vi "YCursorSlider.vi"(5 "Current Trans":u16, 6 "Force Include Focus?":bool=TRUE, 7 "Cursor\nHold-off":dbl, 8 "Dual XDCR Settings":T1 {"XDCR Settings"."UT340 Controls"."Low Pass Filter (MHz)" min=-6 max=60 step=1; "XDCR Settings"."UT340 Controls"."High Pass Filter (MHz)" min=1 max=20 step=1; "XDCR Settings"."UT340 Controls"."Rep Rate (Hz)" min=20 step=1; "XDCR Settings"."UT340 Controls"."Pulse Width (ns)" min=100.0 max=250.0 step=2.0; "XDCR Settings"."UT340 Controls"."Voltage" min=100 max=250 step=2; "XDCR Settings"."UT340 Controls"."PC Gain (dB)" min=2 max=72; "XDCR Settings"."UT340 Controls"."PE Gain (dB)" min=-6 max=60 step=1; "XDCR Settings"."JSR Complete"."JSR Trigger Settings"."PRF (Hz)" items=["100 Hz"=0.1, "200 Hz"=0.2, "400 Hz"=0.4, "600 Hz"=0.6, "800 Hz"=0.8, "1000 Hz"=1.0, "1250 Hz"=1.25, "1500 Hz"=1.5, "1750 Hz"=1.75, "2000 Hz"=2.0, "2500 Hz"=2.5, "3000 Hz"=3.0, "3500 Hz"=3.5, "4000 Hz"=4.0, "4500 Hz"=4.5, "5000 Hz"=5.0]; "XDCR Settings"."JSR Complete"."JSR Trigger Settings"."Trigger Source" items=["Internal", "External"]; "XDCR Settings"."JSR Complete"."JSR Trigger Settings"."External Trigger Limit" items=["No Limit", "5 kHz"]; "XDCR Settings"."JSR Complete"."JSR Receive Settings"."Gain (dB)" min=-13 max=66 step=1; "XDCR Settings"."JSR Complete"."JSR Receive Settings"."Low Pass Filter" items=["5 MHz"=5, "10 MHz"=10, "15 MHz"=15, "22.5 MHz"=22, "35 MHz"=35, "50 MHz"=50]; "XDCR Settings"."JSR Complete"."JSR Receive Settings"."High Pass Filter" items=["DC"=0, "1 MHz"=1000, "2.5 MHz"=2500, "5 MHz"=5000, "7.5 MHz"=7500, "12.5 MHz"=12500]; "XDCR Settings"."JSR Complete"."JSR Receive Settings"."Receiver Mode" items=["Echo", "Through"]; "XDCR Settings"."JSR Complete"."JSR Pulse Settings"."Pulser Voltage (V)" items=["100"=100, "125"=125, "150"=150, "175"=175, "200"=200, "225"=225, "250"=250, "275"=275, "300"=300, "325"=325, "350"=350, "375"=375, "400"=400, "425"=425, "450"=450, "475"=475]; "XDCR Settings"."JSR Complete"."JSR Pulse Settings"."Pulser Impedance" items=["High z", "Low z"]; "XDCR Settings"."JSR Complete"."JSR Pulse Settings"."Pulse Energy Level" items=["0 (Minimum)", "1", "2", "3 (Maximum)"]; "XDCR Settings"."JSR Complete"."JSR Pulse Settings"."Damping" items=["331 Ohms"=331, "198 Ohms"=198, "142 Ohms"=142, "110 Ohms"=110, "92 Ohms"=92, "77 Ohms"=77, "67 Ohms"=67, "59 Ohms"=59, "52 Ohms"=52, "47 Ohms"=47, "43 Ohms"=43, "39 Ohms"=39, "37 Ohms"=37, "34 Ohms"=34, "32 Ohms"=32, "30 Ohms"=30]; "XDCR Settings"."Panametrics Settings"."FINE ATTENUATION" items=["00.0", "00.5", "01.0", "01.5", "02.0", "02.5", "03.0", "03.5", "04.0", "04.5", "05.0", "05.5", "06.0", "06.5", "07.0", "07.5", "08.0", "08.5", "09.0", "09.5", "10.0", "10.5", "11.0", "11.5", "12.0", "12.5", "13.0", "13.5", "14.0", "14.5", "15.0", "15.5"]; "XDCR Settings"."Panametrics Settings"."COARSE ATTENUATION" items=["00.0", "10.0", "20.0", "30.0", "40.0", "50.0"]; "XDCR Settings"."Panametrics Settings"."GAIN (db)" items=["26.0", "40.0", "54.0"]; "XDCR Settings"."Panametrics Settings"."PRF (KHz)" items=["XREMT", "EXBNC", "0.200", "0.500", "1.000", "2.000", "5.000", "10.00", "20.00"]; "XDCR Settings"."Panametrics Settings"."MODE" items=["P/ E", "THRU", "RPP", "EXT_PLSR"]; "XDCR Settings"."Panametrics Settings"."LP FILT (MHz)" items=["20", "50", "100", "200"]; "XDCR Settings"."Panametrics Settings"."HP FILT (KHz)" items=["1", "1000", "3000", "10000"]; "XDCR Settings"."Panametrics Settings"."DAMPING (Ohm)" items=["7", "10", "16", "20", "26", "30", "40", "50"]; "XDCR Settings"."Panametrics Settings"."ENERGY (uJ)" items=["1", "2", "4", "8", "16", "32"]; "XDCR Settings"."Daxsonics Settings"."Freq (MHz)" items=["4"=4, "5"=5, "6"=6, "8"=8, "10"=10, "12"=12, "14"=14, "15"=15, "16"=16, "17"=17, "18"=18, "20"=20, "25"=25, "30"=30, "35"=35, "40"=40, "45"=45, "50"=50]; "XDCR Settings"."Daxsonics Settings"."Voltage (V)" items=["0"=0, "5"=5, "10"=10, "15"=15, "20"=20, "25"=25, "30"=30, "35"=35, "40"=40, "45"=45, "50"=50, "55"=55, "60"=60, "65"=65, "70"=70, "75"=75, "80"=80, "85"=85, "90"=90, "95"=95, "100"=100, "110"=110, "120"=120, "130"=130, "140"=140, "150"=150, "160"=160, "170"=170, "180"=180, "190"=190]; "XDCR Settings"."Daxsonics Settings"."Gain (dB)" items=["22"=22, "25"=25, "28"=28, "31"=31, "34"=34, "37"=37, "40"=40, "43"=43, "46"=46, "49"=49, "52"=52, "55"=55, "58"=58, "61"=61, "64"=64, "67"=67]; "XDCR Settings"."Digitizer Settings"."Additional dig delay (ms)" format="%.2f"; "XDCR Settings"."Digitizer Settings"."Time scale per Div" items=["100 ns"=0.1, "200 ns"=0.2, "500 ns"=0.5, "1 micros"=1.0, "2 micros"=2.0, "5 micros"=5.0, "10 micros"=10.0, "20 micros"=20.0, "50 micros"=50.0, "100 micros"=100.0, "200 micros"=200.0, "500 micros"=500.0, "1 ms"=1000.0, "2 ms"=2000.0, "5 ms"=5000.0, "10 ms"=10000.0, "20 ms"=20000.0, "50 ms"=50000.0, "100 ms"=100000.0, "200 ms"=200000.0]; "XDCR Settings"."Digitizer Settings"."RF data Sampling"."rf points per line" min=1; "XDCR Settings"."Digitizer Settings"."RF data Sampling"."Ref Delay (ms)" format="%.2f"}, 9 "CtlRef":refnum<vi>) -> (1 "Z Scan Size":dbl, 2 "Dual XDCR Settings out":T1 {"XDCR Settings"."UT340 Controls"."Low Pass Filter (MHz)" min=-6 max=60 step=1; "XDCR Settings"."UT340 Controls"."High Pass Filter (MHz)" min=1 max=20 step=1; "XDCR Settings"."UT340 Controls"."Rep Rate (Hz)" min=20 step=1; "XDCR Settings"."UT340 Controls"."Pulse Width (ns)" min=100.0 max=250.0 step=2.0; "XDCR Settings"."UT340 Controls"."Voltage" min=100 max=250 step=2; "XDCR Settings"."UT340 Controls"."PC Gain (dB)" min=2 max=72; "XDCR Settings"."UT340 Controls"."PE Gain (dB)" min=-6 max=60 step=1; "XDCR Settings"."JSR Complete"."JSR Trigger Settings"."PRF (Hz)" items=["100 Hz"=0.1, "200 Hz"=0.2, "400 Hz"=0.4, "600 Hz"=0.6, "800 Hz"=0.8, "1000 Hz"=1.0, "1250 Hz"=1.25, "1500 Hz"=1.5, "1750 Hz"=1.75, "2000 Hz"=2.0, "2500 Hz"=2.5, "3000 Hz"=3.0, "3500 Hz"=3.5, "4000 Hz"=4.0, "4500 Hz"=4.5, "5000 Hz"=5.0]; "XDCR Settings"."JSR Complete"."JSR Trigger Settings"."Trigger Source" items=["Internal", "External"]; "XDCR Settings"."JSR Complete"."JSR Trigger Settings"."External Trigger Limit" items=["No Limit", "5 kHz"]; "XDCR Settings"."JSR Complete"."JSR Receive Settings"."Gain (dB)" min=-13 max=66 step=1; "XDCR Settings"."JSR Complete"."JSR Receive Settings"."Low Pass Filter" items=["5 MHz"=5, "10 MHz"=10, "15 MHz"=15, "22.5 MHz"=22, "35 MHz"=35, "50 MHz"=50]; "XDCR Settings"."JSR Complete"."JSR Receive Settings"."High Pass Filter" items=["DC"=0, "1 MHz"=1000, "2.5 MHz"=2500, "5 MHz"=5000, "7.5 MHz"=7500, "12.5 MHz"=12500]; "XDCR Settings"."JSR Complete"."JSR Receive Settings"."Receiver Mode" items=["Echo", "Through"]; "XDCR Settings"."JSR Complete"."JSR Pulse Settings"."Pulser Voltage (V)" items=["100"=100, "125"=125, "150"=150, "175"=175, "200"=200, "225"=225, "250"=250, "275"=275, "300"=300, "325"=325, "350"=350, "375"=375, "400"=400, "425"=425, "450"=450, "475"=475]; "XDCR Settings"."JSR Complete"."JSR Pulse Settings"."Pulser Impedance" items=["High z", "Low z"]; "XDCR Settings"."JSR Complete"."JSR Pulse Settings"."Pulse Energy Level" items=["0 (Minimum)", "1", "2", "3 (Maximum)"]; "XDCR Settings"."JSR Complete"."JSR Pulse Settings"."Damping" items=["331 Ohms"=331, "198 Ohms"=198, "142 Ohms"=142, "110 Ohms"=110, "92 Ohms"=92, "77 Ohms"=77, "67 Ohms"=67, "59 Ohms"=59, "52 Ohms"=52, "47 Ohms"=47, "43 Ohms"=43, "39 Ohms"=39, "37 Ohms"=37, "34 Ohms"=34, "32 Ohms"=32, "30 Ohms"=30]; "XDCR Settings"."Panametrics Settings"."FINE ATTENUATION" items=["00.0", "00.5", "01.0", "01.5", "02.0", "02.5", "03.0", "03.5", "04.0", "04.5", "05.0", "05.5", "06.0", "06.5", "07.0", "07.5", "08.0", "08.5", "09.0", "09.5", "10.0", "10.5", "11.0", "11.5", "12.0", "12.5", "13.0", "13.5", "14.0", "14.5", "15.0", "15.5"]; "XDCR Settings"."Panametrics Settings"."COARSE ATTENUATION" items=["00.0", "10.0", "20.0", "30.0", "40.0", "50.0"]; "XDCR Settings"."Panametrics Settings"."GAIN (db)" items=["26.0", "40.0", "54.0"]; "XDCR Settings"."Panametrics Settings"."PRF (KHz)" items=["XREMT", "EXBNC", "0.200", "0.500", "1.000", "2.000", "5.000", "10.00", "20.00"]; "XDCR Settings"."Panametrics Settings"."MODE" items=["P/ E", "THRU", "RPP", "EXT_PLSR"]; "XDCR Settings"."Panametrics Settings"."LP FILT (MHz)" items=["20", "50", "100", "200"]; "XDCR Settings"."Panametrics Settings"."HP FILT (KHz)" items=["1", "1000", "3000", "10000"]; "XDCR Settings"."Panametrics Settings"."DAMPING (Ohm)" items=["7", "10", "16", "20", "26", "30", "40", "50"]; "XDCR Settings"."Panametrics Settings"."ENERGY (uJ)" items=["1", "2", "4", "8", "16", "32"]; "XDCR Settings"."Daxsonics Settings"."Freq (MHz)" items=["4"=4, "5"=5, "6"=6, "8"=8, "10"=10, "12"=12, "14"=14, "15"=15, "16"=16, "17"=17, "18"=18, "20"=20, "25"=25, "30"=30, "35"=35, "40"=40, "45"=45, "50"=50]; "XDCR Settings"."Daxsonics Settings"."Voltage (V)" items=["0"=0, "5"=5, "10"=10, "15"=15, "20"=20, "25"=25, "30"=30, "35"=35, "40"=40, "45"=45, "50"=50, "55"=55, "60"=60, "65"=65, "70"=70, "75"=75, "80"=80, "85"=85, "90"=90, "95"=95, "100"=100, "110"=110, "120"=120, "130"=130, "140"=140, "150"=150, "160"=160, "170"=170, "180"=180, "190"=190]; "XDCR Settings"."Daxsonics Settings"."Gain (dB)" items=["22"=22, "25"=25, "28"=28, "31"=31, "34"=34, "37"=37, "40"=40, "43"=43, "46"=46, "49"=49, "52"=52, "55"=55, "58"=58, "61"=61, "64"=64, "67"=67]; "XDCR Settings"."Digitizer Settings"."Additional dig delay (ms)" format="%.2f"; "XDCR Settings"."Digitizer Settings"."Time scale per Div" items=["100 ns"=0.1, "200 ns"=0.2, "500 ns"=0.5, "1 micros"=1.0, "2 micros"=2.0, "5 micros"=5.0, "10 micros"=10.0, "20 micros"=20.0, "50 micros"=50.0, "100 micros"=100.0, "200 micros"=200.0, "500 micros"=500.0, "1 ms"=1000.0, "2 ms"=2000.0, "5 ms"=5000.0, "10 ms"=10000.0, "20 ms"=20000.0, "50 ms"=50000.0, "100 ms"=100000.0, "200 ms"=200000.0]; "XDCR Settings"."Digitizer Settings"."RF data Sampling"."rf points per line" min=1; "XDCR Settings"."Digitizer Settings"."RF data Sampling"."Ref Delay (ms)" format="%.2f"})   [LabVIEW 2022 SP3]
uses:
  ScanningControl/DualXDCR/Dual XDCR Complete Settings.ctl
  ScanningControl/DualXDCR/XDCRSettings.ctl
  ScanningControl/Pulsers/Daxsonics/-DaxSubroutines/Dax_Control_Cluster.ctl
  ScanningControl/Pulsers/Panametrics/Pana5900.ctl
  ScanningControl/Pulsers/JSR/Controls/JSR Complete.ctl
  ScanningControl/Pulsers/JSR/Controls/JSR Pulse.ctl
  ScanningControl/Pulsers/JSR/Controls/Damping.ctl
  ScanningControl/Pulsers/JSR/Controls/Energy.ctl
  ScanningControl/Pulsers/JSR/Controls/Z.ctl
  ScanningControl/Pulsers/JSR/Controls/Volt.ctl
  ScanningControl/Pulsers/JSR/Controls/JSR Recieve.ctl
  ScanningControl/Pulsers/JSR/Controls/Mode.ctl
  ScanningControl/Pulsers/JSR/Controls/HPF.ctl
  ScanningControl/Pulsers/JSR/Controls/LPF.ctl
  ScanningControl/Pulsers/JSR/Controls/Gain.ctl
  ScanningControl/Pulsers/JSR/Controls/JSR Trigger.ctl
  ScanningControl/Pulsers/JSR/Controls/Trig Limit.ctl
  ScanningControl/Pulsers/JSR/Controls/Trig Source.ctl
  ScanningControl/Pulsers/JSR/Controls/PRF.ctl
  ScanningControl/Pulsers/UTEX/Controls/UTEX Controls.ctl
  <vilib>/Analysis/baseanly.llb/Mean (DBL).vi
  Misc Programs/MathOperations/ModuloFraction.vi
  <vilib>/Analysis/NI_AALBase.lvlib
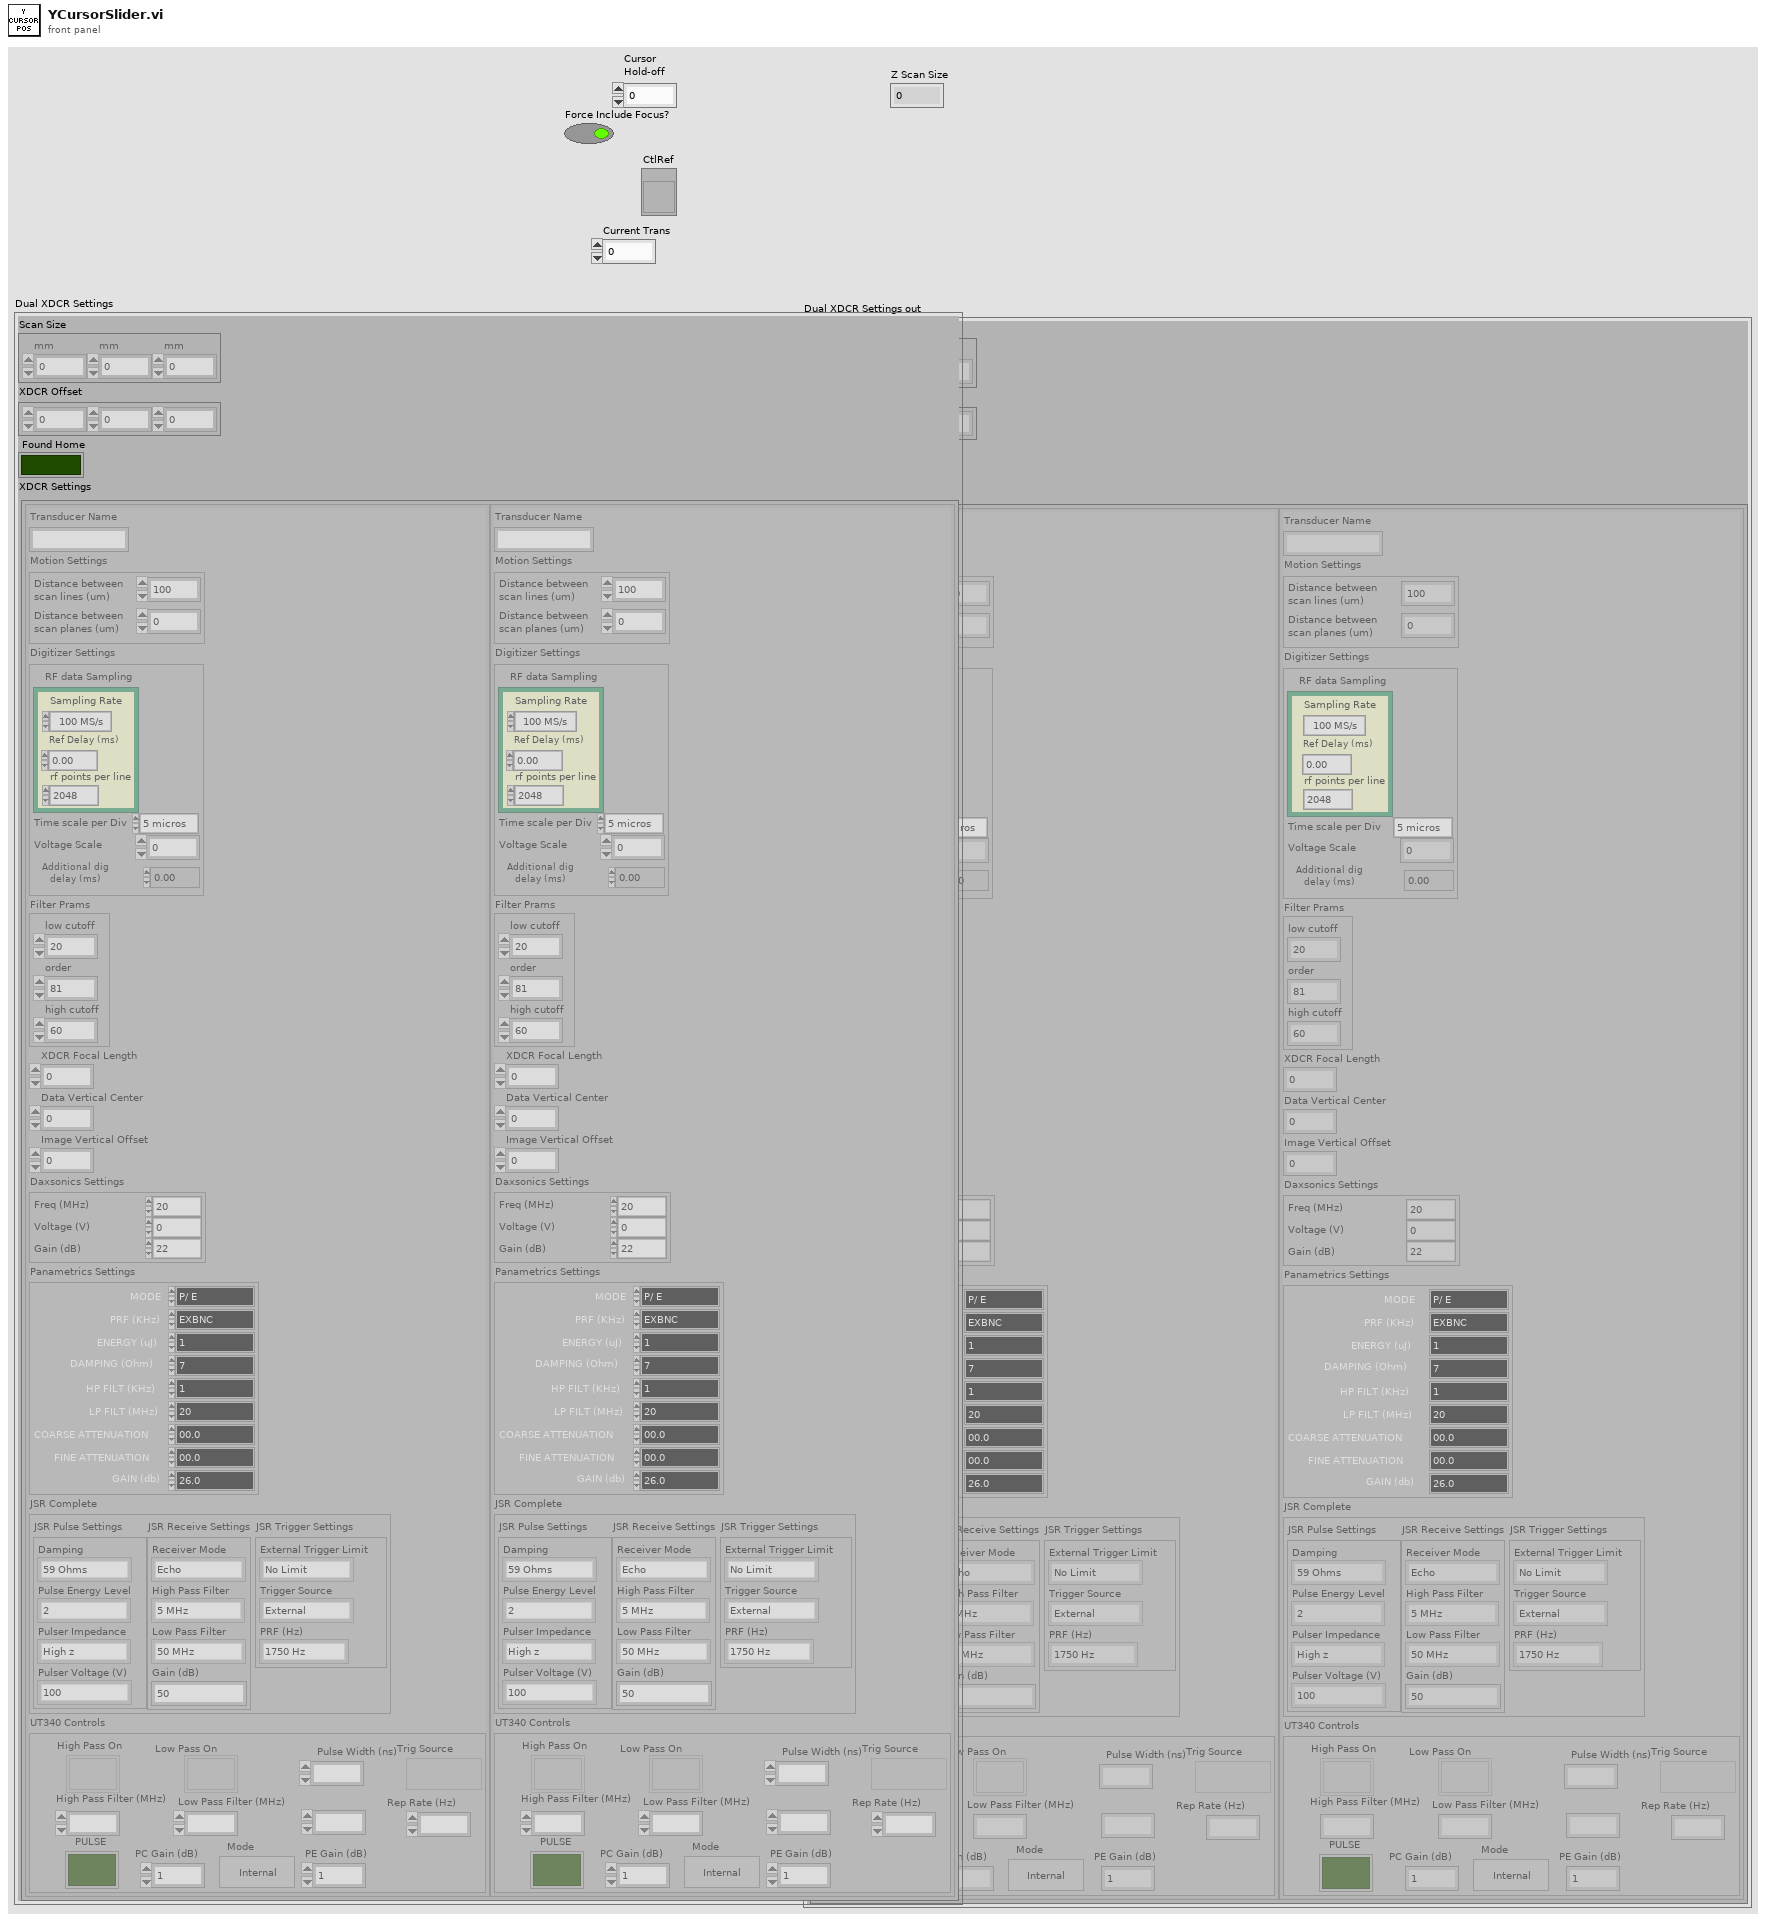
[diagram p1: front panel]
types:
  T1 = typedef "Dual XDCR Complete Settings.ctl" = cluster{"Scan Size":dbl[], "XDCR Offset":dbl[], "Found Home":bool, "XDCR Settings":T2[]}
  T2 = typedef "XDCRSettings.ctl" = cluster{"Transducer Name":string, "Motion Settings":cluster{"Distance between\nscan lines (um)":sgl, "Distance between\nscan planes (um)":sgl}, "Digitizer Settings":cluster{"RF data Sampling":cluster{"Sampling Rate":dbl, "Ref Delay (ms)":dbl, "rf points per line":i32}, "Time scale per Div":dbl, "Voltage Scale":dbl, "Additional dig delay (ms)":dbl}, "Filter Prams":cluster{"low cutoff":i32, "order":i32, "high cutoff":i32}, "XDCR Focal Length":dbl, "Data Vertical Center":dbl, "Image Vertical Offset":dbl, "Daxsonics Settings":T3, "Panametrics Settings":T4, "JSR Complete":T5, "UT340 Controls":T20}
  T3 = typedef "Dax_Control_Cluster.ctl" = cluster{"Freq (MHz) ":u16, "Voltage (V)":u16, "Gain (dB)":u16}
  T4 = typedef "Pana5900.ctl" = cluster{"ENERGY (uJ)":u16, "DAMPING (Ohm)":u16, "HP FILT (KHz) ":u16, "LP FILT (MHz)":u16, "MODE":u16, "PRF (KHz)":u16, "GAIN (db)":u16, "COARSE ATTENUATION":u16, "FINE ATTENUATION":u16}
  T5 = typedef "JSR Complete.ctl" = cluster{"JSR Pulse Settings":T6, "JSR Receive Settings":T11, "JSR Trigger Settings":T16}
  T6 = typedef "JSR Pulse.ctl" = cluster{"Damping":T7, "Pulse Energy Level":T8, "Pulser Impedance":T9, "Pulser Voltage (V)":T10}
  T7 = typedef "Damping.ctl" = i16
  T8 = typedef "Energy.ctl" = u16
  T9 = typedef "Z.ctl" = u16
  T10 = typedef "Volt.ctl" = i16
  T11 = typedef "JSR Recieve.ctl" = cluster{"Receiver Mode":T12, "High Pass Filter":T13, "Low Pass Filter":T14, "Gain (dB)":T15}
  T12 = typedef "Mode.ctl" = i8
  T13 = typedef "HPF.ctl" = u16
  T14 = typedef "LPF.ctl" = u16
  T15 = typedef "Gain.ctl" = i8
  T16 = typedef "JSR Trigger.ctl" = cluster{"External Trigger Limit":T17, "Trigger Source":T18, "PRF (Hz)":T19}
  T17 = typedef "Trig Limit.ctl" = i8
  T18 = typedef "Trig Source.ctl" = i8
  T19 = typedef "PRF.ctl" = dbl
  T20 = typedef "UTEX Controls.ctl" = cluster{"High Pass On":bool, "High Pass Filter (MHz)":i16, "Low Pass On":bool, "Low Pass Filter (MHz)":i16, "PE Gain (dB)":i16, "Voltage":i16, "Pulse Width (ns)":dbl, "Mode":bool, "PC Gain (dB)":i16, "Trig Source":bool, "Rep Rate (Hz)":i16, "PULSE":bool}
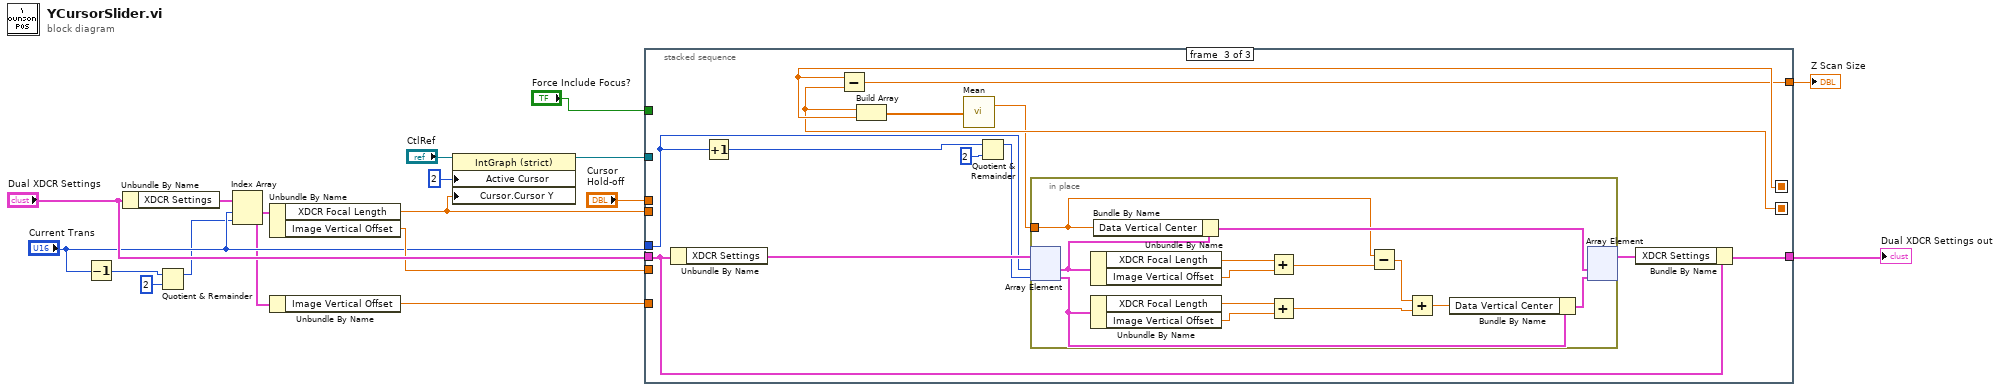
[diagram p0: block diagram]
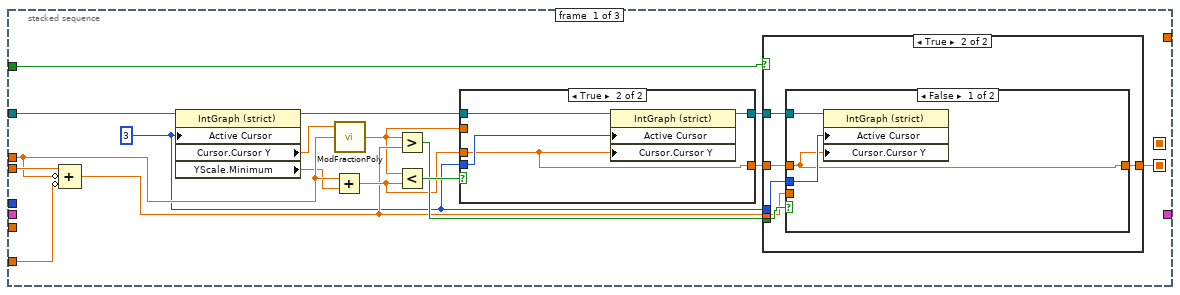
[diagram p2: hidden frame]
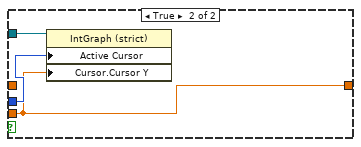
[diagram p4: hidden frame]
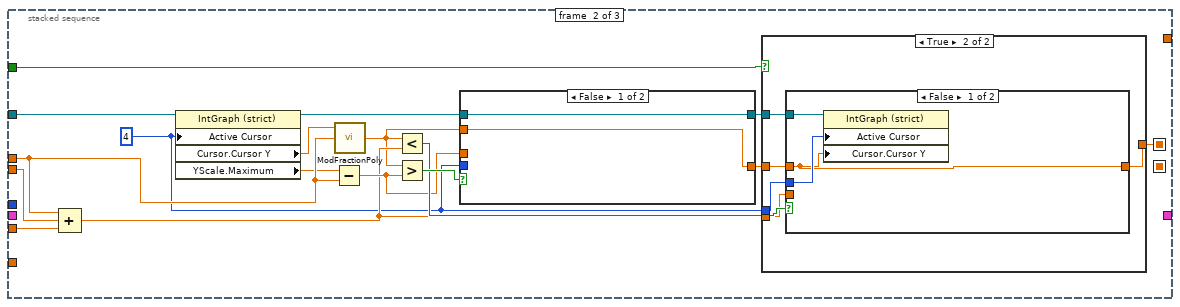
[diagram p6: hidden frame]
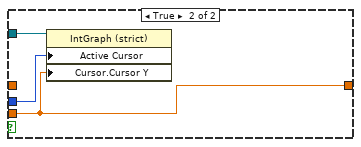
[diagram p8: hidden frame]
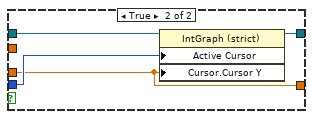
[diagram p9: hidden frame]
diagram:
  n1 = Decrement(x="Current Trans") -> (x-1=w1:u16)
  n2 = Unbundle By Name("Dual XDCR Settings") -> ("XDCR Settings"=w12:T2[])
  n3 = Quotient & Remainder(x=w1, y=u32 2) -> (x-y*floor(x/y)=w4:u32)  [unwired: 1 out]
  n4 = Index Array(array=w12, index #1="Current Trans", index #2=w4) -> (element #1=w13:T2, element #2=w3:T2)
  n5 = Unbundle By Name(w13) -> ("XDCR Focal Length"=w10:dbl, "Image Vertical Offset"=w7:dbl)
  n6 = Unbundle By Name(w3) -> ("Image Vertical Offset"=w2:dbl)
  n7 = property on="Property Node" class="IntGraph (strict)"(reference="CtlRef", "Active Cursor"=u32 2, "Cursor.Cursor Y"=w10) -> (reference out=w15:refnum<vi>)  [unwired: 1 in, 1 out]
  n8 = stacked-sequence {
    seq-local: [w33 _ _] -> [_ _ w94]
    seq-local: [_ w69 _] -> [_ _ w95]
    tunnel: w15 -> [w25 w61 _]
    tunnel: "Dual XDCR Settings" -> [_ _ w97]
    tunnel: "Current Trans" -> [_ _ w102]
    tunnel: w10 -> [w32 w68 _]
    tunnel: "Cursor\nHold-off" -> [w28 w65 _]
    tunnel: [_ _ w93] -> w17
    tunnel: [_ _ w92] -> w9
    tunnel: "Force Include Focus?" -> [w20 w56 _]
    tunnel: w7 -> [_ w55 _]
    tunnel: w2 -> [w19 _ _]
    frame #0 {
      w27 = u32 3 ("Active Cursor")
      n9 = Compound Arithmetic op=ADD(w32, invert w28, invert w19) -> (w30:dbl)
      n10 = property on="Property Node" class="IntGraph (strict)"(reference=w25, "Active Cursor"=w27) -> (reference out=w24:refnum<vi>, "Cursor.Cursor Y"=w26:dbl, "YScale.Minimum"=w23:dbl)  [unwired: 1 in, 1 out]
      n11 = Add(x=w28, y=w23) -> (x+y=w31:dbl)
      n12 = call-poly "ModFractionPoly.vi"("Modulo Fraction"=w28, "Input"=w26) -> ("Output"=w29:dbl)  [unwired: 1 in]
      n13 = Greater?(x=w29, y=w30) -> (0:w34:bool)
      n14 = Less?(x=w29, y=w31) -> (x < y?=w35:bool)
      n15 = case shown="True" w35 {
        tunnel: w24 -> [w49 w54]
        tunnel: [w50 w51] -> w22
        tunnel: w29 -> [w50 _]
        tunnel: w27 -> [_ w53]
        tunnel: w31 -> [_ w51]
        tunnel: [w49 w52] -> w21
        frame False {
        }
        frame True {
          n16 = property on="Property Node" class="IntGraph (strict)"(reference=w54, "Active Cursor"=w53, "Cursor.Cursor Y"=w51) -> (reference out=w52:refnum<vi>)  [unwired: 1 in, 1 out]
        }
      }
      n17 = case shown="True" w20 {
        tunnel: w34 -> [_ w42]
        tunnel: [w36 w41] -> w33
        tunnel: w30 -> [_ w40]
        tunnel: w27 -> [_ w39]
        tunnel: w22 -> [w36 w38]
        tunnel: w21 -> [_ w37]
        frame False {
        }
        frame True {
          n18 = case shown="False" w42 {
            tunnel: w37 -> [w45 w48]
            tunnel: w39 -> [w44 w47]
            tunnel: w40 -> [_ w46]
            tunnel: w38 -> [w43 _]
            tunnel: [w43 w46] -> w41
            frame False {
              n19 = property on="Property Node" class="IntGraph (strict)"(reference=w45, "Active Cursor"=w44, "Cursor.Cursor Y"=w43) -> ()  [unwired: 1 in, 2 out]
            }
            frame True {
              n20 = property on="Property Node" class="IntGraph (strict)"(reference=w48, "Active Cursor"=w47, "Cursor.Cursor Y"=w46) -> ()  [unwired: 1 in, 2 out]
            }
          }
        }
      }
    }
    frame #1 {
      w63 = u32 4 ("Active Cursor")
      n21 = Compound Arithmetic op=ADD(w65, w68, w55) -> (w66:dbl)
      n22 = property on="Property Node" class="IntGraph (strict)"(reference=w61, "Active Cursor"=w63) -> (reference out=w62:refnum<vi>, "Cursor.Cursor Y"=w60:dbl, "YScale.Maximum"=w59:dbl)  [unwired: 1 in, 1 out]
      n23 = Subtract(x=w59, y=w65) -> (x-y=w67:dbl)
      n24 = call-poly "ModFractionPoly.vi"("Modulo Fraction"=w65, "Input"=w60) -> ("Output"=w64:dbl)  [unwired: 1 in]
      n25 = Less?(x=w64, y=w66) -> (x < y?=w70:bool)
      n26 = Greater?(x=w64, y=w67) -> (0:w71:bool)
      n27 = case shown="False" w71 {
        tunnel: w62 -> [w85 w90]
        tunnel: [w86 w88] -> w58
        tunnel: w64 -> [w86 _]
        tunnel: w63 -> [_ w89]
        tunnel: w67 -> [_ w88]
        tunnel: [w85 w87] -> w57
        frame False {
        }
        frame True {
          n28 = property on="Property Node" class="IntGraph (strict)"(reference=w90, "Active Cursor"=w89, "Cursor.Cursor Y"=w88) -> (reference out=w87:refnum<vi>)  [unwired: 1 in, 1 out]
        }
      }
      n29 = case shown="True" w56 {
        tunnel: w70 -> [_ w78]
        tunnel: [w72 w77] -> w69
        tunnel: w66 -> [_ w76]
        tunnel: w63 -> [_ w75]
        tunnel: w58 -> [w72 w74]
        tunnel: w57 -> [_ w73]
        frame False {
        }
        frame True {
          n30 = case shown="False" w78 {
            tunnel: w73 -> [w81 w84]
            tunnel: w75 -> [w80 w83]
            tunnel: w76 -> [_ w82]
            tunnel: w74 -> [w79 _]
            tunnel: [w79 w82] -> w77
            frame False {
              n31 = property on="Property Node" class="IntGraph (strict)"(reference=w81, "Active Cursor"=w80, "Cursor.Cursor Y"=w79) -> ()  [unwired: 1 in, 2 out]
            }
            frame True {
              n32 = property on="Property Node" class="IntGraph (strict)"(reference=w84, "Active Cursor"=w83, "Cursor.Cursor Y"=w82) -> ()  [unwired: 1 in, 2 out]
            }
          }
        }
      }
    }
    frame #2 {
      n33 = Unbundle By Name(w97) -> ("XDCR Settings"=w103:T2[])
      n34 = Increment(x=w102) -> (x+1=w101:u16)
      n35 = Subtract(x=w95, y=w94) -> (x-y=w92:dbl)
      n36 = Build Array(w94, w95) -> (w96:dbl[])
      n37 = call-poly <vilib>:"Mean.vi"("X"=w96) -> ("mean"=w91:dbl)  [unwired: 1 out]
      n38 = Quotient & Remainder(x=w101, y=u32 2) -> (x-y*floor(x/y)=w99:u32)  [unwired: 1 out]
      n39 = in-place {
        in-place-border: w91 -> [w111]
        n40 = in-place-array #1(w103, w102, w99) -> (w115:T2, w106:T2)
        n41 = Unbundle By Name(w115) -> ("XDCR Focal Length"=w114:dbl, "Image Vertical Offset"=w113:dbl)
        n42 = Unbundle By Name(w106) -> ("XDCR Focal Length"=w107:dbl, "Image Vertical Offset"=w110:dbl)
        n43 = Bundle By Name(cluster=w115, "Data Vertical Center"=w111) -> (w116:T2)
        n44 = Add(x=w114, y=w113) -> (x+y=w112:dbl)
        n45 = Add(x=w107, y=w110) -> (x+y=w109:dbl)
        n46 = Subtract(x=w111, y=w112) -> (x-y=w104:dbl)
        n47 = Add(x=w104, y=w109) -> (x+y=w108:dbl)
        n48 = Bundle By Name(cluster=w106, "Data Vertical Center"=w108) -> (w105:T2)
        n49 = in-place-array #1(w116, w105) -> (w98:T2[])  [unwired: 2 out]
      }
      n50 = Bundle By Name(cluster=w97, "XDCR Settings"=w98) -> (w93:T1)
    }
  }
  "Dual XDCR Settings out" <- w17
  "Z Scan Size" <- w9
